vi "LVDimInterface.VI-Tree.vi"   [LabVIEW 2014, in "LVDimInterface.lvlib"]
doc: "This is a VI-Tree containing all VIs of the LabVIEW-DIM interface. For more information, have a look at the documentation of the library \"LVDimInterface.lvlib\"\n\nHistory: 27-OCT-2008, Dietrich Beck\n\nCopyright (C)\nGesellschaft für Schwerionenforschung, GSI\nPlanckstr. 1\n64291 Darmstadt\nGermany\n\nContact: D.Beck@gsi.de \n\nThis program is free software; you can redistribute it and/or modify it under the terms of the GNU General Public License as published by the Free Software Foundation; either version 2 of the license, or (at your option) any later version.\n\nThis program is distributed in the hope that it will be useful, but WITHOUT ANY WARRANTY; without even the implied warranty of MERCHANTABILITY or FITNESS FOR A PARTICULAR PURPOSE. See the GNU General License for more details (http://www.gnu.org).\n\nGesellschaft für Schwerionenforschung, GSI\nPlanckstr. 1, 64291 Darmstadt, Germany\nFor all questions and ideas contact D. Beck.\nLast update: 16-DEC-2005"
uses:
  LVDimInterface.lvlib
  LVDimInterface.queue type.ctl
  LVDimInterface.dic_info_service_notifier.vi
  LVDimInterface.dis_add_command_queue.vi
panel:
  # "SEE DIAGRAM\nFOR VI TREE."
types:
  T1 = typedef "LVDimInterface.lvlib/LVDimInterface.queue type.ctl" = refnum<queue>
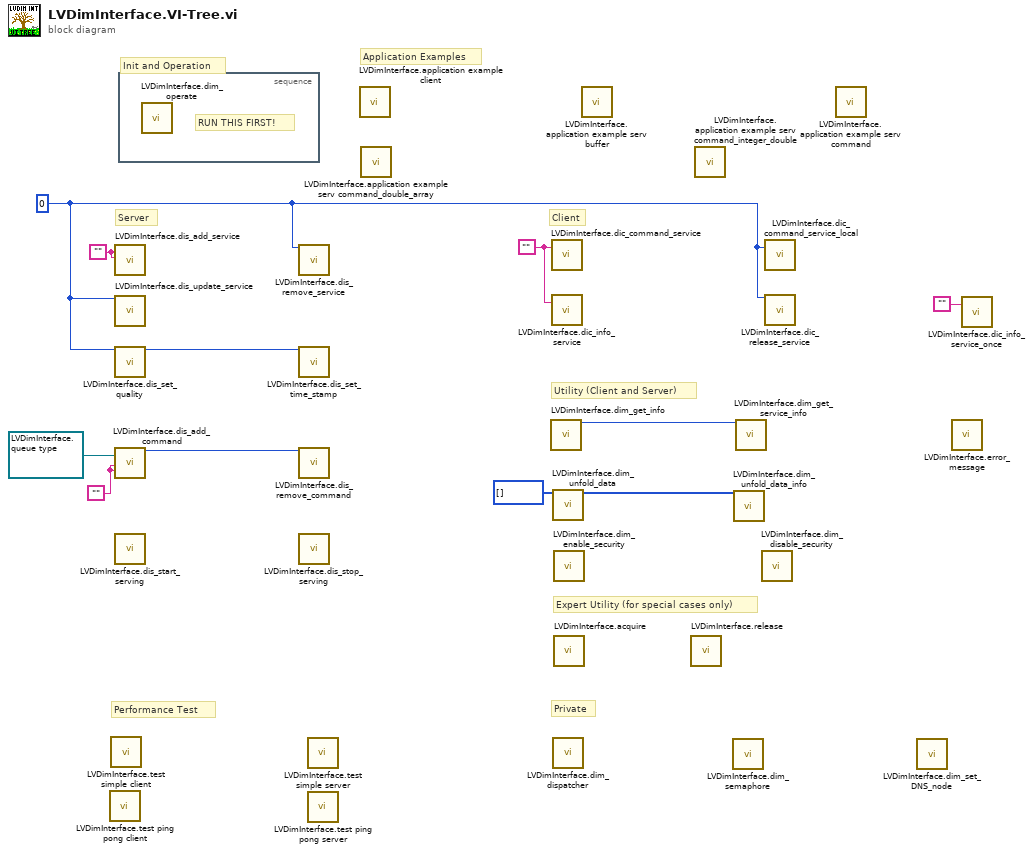
[diagram p0: block diagram]
diagram:
  w1 = "" ("commandName")
  w11 = "" ("commandName")
  w9 = 0 ("my_serviceID")
  w2 = "" ("serviceName")
  # "Expert Utility (for special cases only)"
  # "Init and Operation"
  # "Private"
  # "Performance Test"
  # "Utility (Client and Server)"
  # "Client"
  # "Server"
  # "Application Examples"
  n1 = call "LVDimInterface.test ping pong client.vi"() -> ()  [unwired: 1 in]
  n2 = call "LVDimInterface.test simple client.vi"() -> ()  [unwired: 1 in]
  n3 = call "LVDimInterface.dis_add_service.vi"("serviceName"=w2, "typeDescriptor"=w2) -> ()  [unwired: 16 in, 2 out]
  n4 = call "LVDimInterface.dis_update_service.vi"("my_serviceID"=w9) -> ()  [unwired: 16 in, 3 out]
  n5 = call "LVDimInterface.dis_set_quality.vi"("my_serviceID"=w9) -> ("my_serviceID (out)"=w8:i32)  [unwired: 17 in, 1 out]
  n6 = call-poly "LVDimInterface.dis_add_command.vi"("queueRef"=T1 refnum, "commandName"=w1, "typeDescriptor"=w1) -> ("commandID"=w5:i32)  [unwired: 15 in, 1 out]
  n7 = call "LVDimInterface.dis_start_serving.vi"() -> ()  [unwired: 18 in, 2 out]
  n8 = stacked-sequence {
    frame #0 {
      # "RUN THIS FIRST!"
      n9 = call "LVDimInterface.dim_operate.vi"() -> ()  [unwired: 20 in]
    }
  }
  n10 = call "LVDimInterface.dis_remove_service.vi"("my_serviceID"=w9) -> ()  [unwired: 18 in, 1 out]
  n11 = call "LVDimInterface.dis_set_time_stamp.vi"("my_serviceID"=w8) -> ()  [unwired: 17 in, 2 out]
  n12 = call "LVDimInterface.dis_remove_command.vi"("commandID"=w5) -> ()  [unwired: 18 in, 1 out]
  n13 = call "LVDimInterface.dis_stop_serving.vi"() -> ()  [unwired: 19 in, 1 out]
  n14 = call "LVDimInterface.test simple server.vi"() -> ()  [unwired: 1 in]
  n15 = call "LVDimInterface.test ping pong server.vi"() -> ()  [unwired: 1 in]
  n16 = call "LVDimInterface.application example client.vi"() -> ()  [unwired: 1 in]
  n17 = call "LVDimInterface.application example serv command_double_array.vi"() -> ()  [unwired: 1 in]
  n18 = call "LVDimInterface.dim_get_info.vi"() -> ("versionNumber"=w7:i32)  [unwired: 13 in, 6 out]
  n19 = call "LVDimInterface.dic_command_service.vi"("commandName"=w11) -> ()  [unwired: 17 in, 2 out]
  n20 = call-poly "LVDimInterface.dic_info_service.vi"("serviceName"=w11) -> ()  [unwired: 17 in, 2 out]
  n21 = call "LVDimInterface.dim_unfold_data.vi"("rawData"=i8[] []) -> ("data"=w3:i8[])  [unwired: 15 in, 3 out]
  n22 = call "LVDimInterface.dim_dispatcher.vi"() -> ()  [unwired: 20 in]
  n23 = call "LVDimInterface.dim_enable_security.vi"() -> ()  [unwired: 19 in, 1 out]
  n24 = call "LVDimInterface.acquire.vi"() -> ()  [unwired: 18 in, 2 out]
  n25 = call "LVDimInterface.application example serv buffer.vi"() -> ()  [unwired: 1 in]
  n26 = call "LVDimInterface.release.vi"() -> ()  [unwired: 19 in, 1 out]
  n27 = call "LVDimInterface.application example serv command_integer_double.vi"() -> ()  [unwired: 1 in]
  n28 = call "LVDimInterface.dim_semaphore.vi"() -> ()  [unwired: 19 in, 1 out]
  n29 = call "LVDimInterface.dim_unfold_data_info.vi"("rawData"=w3) -> ()  [unwired: 8 in, 11 out]
  n30 = call "LVDimInterface.dim_get_service_info.vi"("callBackID"=w7) -> ()  [unwired: 9 in, 10 out]
  n31 = call "LVDimInterface.dim_disable_security.vi"() -> ()  [unwired: 19 in, 1 out]
  n32 = call "LVDimInterface.dic_command_service_local.vi"("commandID"=w9) -> ()  [unwired: 17 in, 2 out]
  n33 = call "LVDimInterface.dic_release_service.vi"("callBackID"=w9) -> ()  [unwired: 18 in, 1 out]
  n34 = call "LVDimInterface.application example serv command.vi"() -> ()  [unwired: 1 in]
  n35 = call "LVDimInterface.dim_set_DNS_node.vi"() -> ()  [unwired: 18 in, 2 out]
  n36 = call "LVDimInterface.error_message.vi"() -> ()  [unwired: 16 in, 4 out]
  n37 = call "LVDimInterface.dic_info_service_once.vi"("serviceName"="") -> ()  [unwired: 15 in, 4 out]
